vi "SubDaqStop.vi"(8 "error in (no error)":errorcluster, 9 "SubQueueIN":refnum<queue>, 10 "MainQueueIN":refnum<queue>, 11 "Data Value Reference IN":refnum<data-value>) -> (0 "error out":errorcluster, 3 "Data Value Reference out":refnum<data-value>)   [LabVIEW 2013]
uses:
  Control/SystemCommand.ctl
  Control/SystemData.ctl
  Control/SignalType.ctl
  Control/SubDaqCommand.ctl
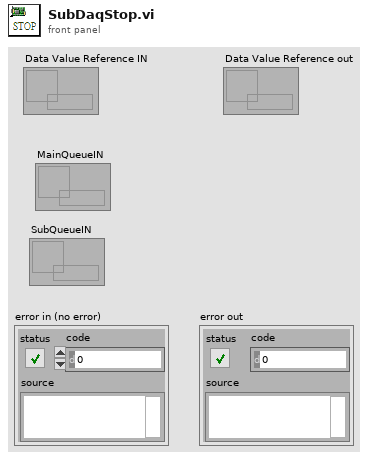
[diagram p1: front panel]
types:
  T1 = typedef "SystemCommand.ctl" = enum16{"None", "Init", "Close", "ShowNumeric", "ShowString", "ShowBool", "SquareNumeric", "ReverseString", "InvertBool", "FFT"}
  T2 = typedef "SystemData.ctl" = cluster{"Numeric":dbl, "String":string, "Boolean":bool, "Frequency":dbl, "Amplitude":dbl, "SignalType":T3, "WaveformArray":waveform(dbl)[], "Reset":bool, "StateString":string, "FFTmagnitudes":cluster{"f0":dbl, "df":dbl, "magnitude":dbl[]}[]}
  T3 = typedef "SignalType.ctl" = enum16{"Sin", "Triangle", "Square"}
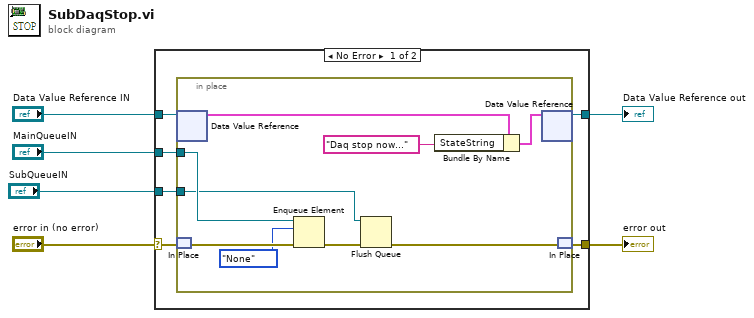
[diagram p0: block diagram]
diagram:
  n1 = case shown="No Error" "error in (no error)" {
    selector: "error in (no error)" -> [w10 w22]
    tunnel: "Data Value Reference IN" -> [w12 w23]
    tunnel: [w11 w23] -> w3
    tunnel: [w9 w22] -> w5
    tunnel: "MainQueueIN" -> [w8 _]
    tunnel: "SubQueueIN" -> [w7 _]
    frame No Error {
      n2 = in-place {
        in-place-border: w8 -> [w20]
        in-place-border: w7 -> [w17]
        n3 = in-place-dvr #1(w12) -> (w14:T2)  [unwired: 1 out]
        n4 = in-place-match #2(w10) -> (w21:errorcluster)
        n5 = Enqueue Element(queue=w20, element=SystemCommand."None" ("Command"), error in (no error)=w21) -> (error out=w18:errorcluster)  [unwired: 1 in, 2 out]
        n6 = Flush Queue(queue=w17, error in (no error)=w18) -> (error out=w16:errorcluster)  [unwired: 2 out]
        n7 = Bundle By Name(cluster=w14, "StateString"="Daq stop now..." ("Message")) -> (w13:T2)
        n8 = in-place-dvr #1(w13) -> (w11:refnum<data-value>)  [unwired: 1 out]
        n9 = in-place-match #2(w16) -> (w9:errorcluster)
      }
    }
    frame Error {
    }
  }
  "error out" <- w5
  "Data Value Reference out" <- w3
